vi "Log.vi"(9 "data":variant, 10 "message":string, 11 "level":T1) -> ()   [LabVIEW 2018, in "GLog.lvlib" / "Registry.lvlib"]
uses:
  Registry.lvlib
  api/Log Levels.ctl
  Registry Actions.ctl
  dependencies/Utilities/Utilities.lvlib
  api/logger_class/Logger.lvclass
  api/GLog.lvlib
panel:
  # "Connector Pane"
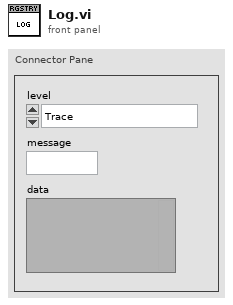
[diagram p1: front panel]
types:
  T1 = typedef "GLog.lvlib/Log Levels.ctl" = enum16{"Trace", "Debug", "Info", "Warning", "Error", "Critical"}
  T2 = typedef "GLog.lvlib/Registry.lvlib/Registry Actions.ctl" = enum16{"Register", "Log", "Enable", "Enable All", "Disable", "Disable All", "Get Enable State", "Get Minimum Log Level", "Set Minimum Log Level", "Set All Minimum Log Level", "Get Logger Info", "Get All Logger Info", "List", "Unregister", "Unregister All", "Shutdown"}
  T3 = typedef "GLog.lvlib/Log Record.ctl" = cluster{"level":T4, "timestamp":timestamp, "call chain":string[], "message":string, "data":variant}
  T4 = typedef "GLog.lvlib/Internal Log Levels.ctl" = enum16{"Trace", "Debug", "Info", "Warning", "Error", "Critical", "Internal"}
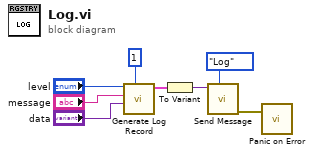
[diagram p0: block diagram]
diagram:
  n1 = call "Generate Log Record.vi"("call chain elements to ignore (0)"=1, "data (null)"="data", "message (\"\")"="message", "log level"="level") -> ("log record"=w2:T3)  [unwired: 7 in]
  n2 = To Variant(anything=w2) -> (Variant=w8:variant)
  n3 = call "Send Message.vi"("action"=Registry_Actions."Log", "send data"=w8) -> ("error out"=w7:errorcluster)  [unwired: 8 in, 1 out]
  n4 = call "Panic on Error.vi"("error in (no error)"=w7) -> ()  [unwired: 3 in]
